vi "LED XControl Scroll.vi"(9 "Single pass?":bool, 10 "LEDDisplay":refnum<vi>, 11 "String":string="The Software is the Instrument     ") -> ()   [LabVIEW 2012, in "LED Display.xctl"]
doc: "This VI will control scrolling the XControl LED and displaying the string on LED Screen"
uses:
  LED Display.xctl
panel:
  # "This is the actual background task VI. It is reentrant and multiple clones of this VI may exist in memory, one for each of the LED XControls."
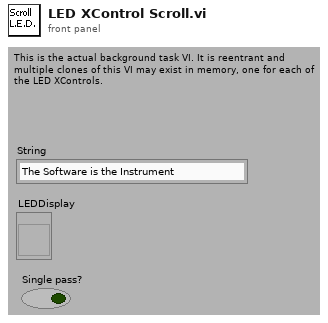
[diagram p1: front panel]
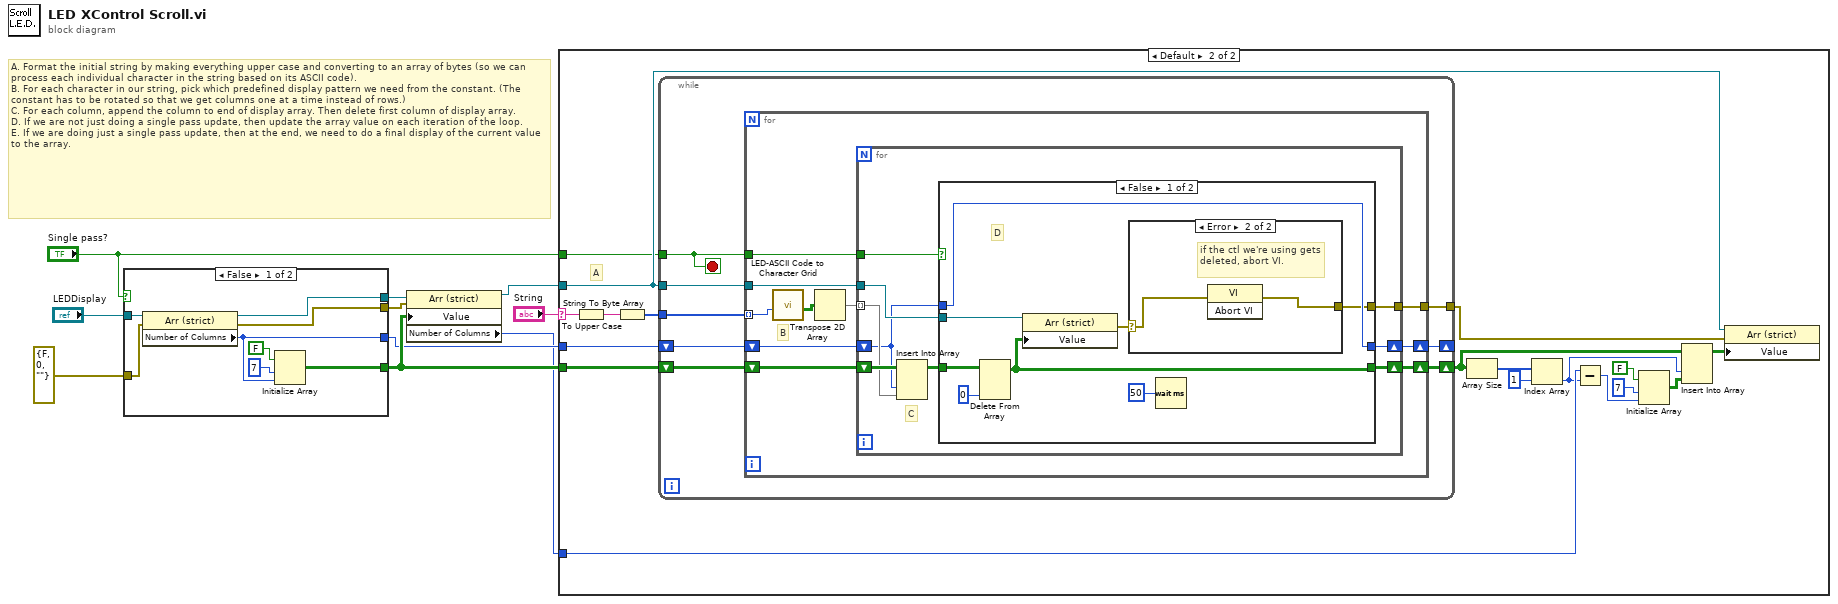
[diagram p0: block diagram]
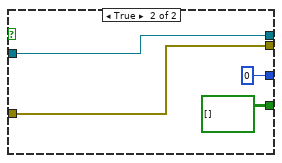
[diagram p2: hidden frame]
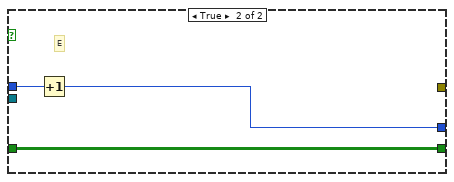
[diagram p5: hidden frame]
diagram:
  # "A. Format the initial string by making everything upper case and converting to an array of bytes (so we can process each individual character in the string based on its ASCII code).\nB. For each character in our string, pick which predefined display pattern we need from the constant. (The constant has to be rotated so that we get columns one at a time instead of rows.)\nC. For each column, append the column to end of display array. Then delete first column of display array.\nD. If we are not just doing a single pass update, then update the array value on each iteration of the loop.\nE. If we are doing just a single pass update, then at the end, we need to do a final display of the current value to the array."
  n1 = case shown="False" "Single pass?" {
    tunnel: "LEDDisplay" -> [w18 w22]
    tunnel: [w17 w22] -> w8
    tunnel: [w16 bool[][] []] -> w7
    tunnel: [w13 u32 0 ("Number of Columns")] -> w4
    tunnel: [w12 w19] -> w2
    tunnel: errorcluster {"status"=FALSE, "code"=0, "source"=""} ("error out") -> [w11 w19]
    frame False {
      n2 = property class="Arr (strict)"(reference=w18, error in=w11) -> (reference out=w17:refnum<vi>, error out=w12:errorcluster, "Number of Columns"=w13:u32)
      n3 = Initialize Array(FALSE ("Boolean"), 7 ("dimension size"), w13) -> (w16:bool[][])
    }
    frame True {
    }
  }
  n4 = property class="Arr (strict)"(reference=w8, error in=w2, "Value"=w7) -> (reference out=w6:refnum<vi>, "Number of Columns"=w3:u32)  [unwired: 1 out]
  n5 = case shown="Default" "String" {
    selector: "String" -> [_ w39]
    tunnel: w6 -> [_ w37]
    tunnel: w7 -> [_ w38]
    tunnel: "Single pass?" -> [_ w36]
    tunnel: w4 -> [_ w35]
    tunnel: w3 -> [_ w32]
    frame "" {
      # "do nothing for empty string."
    }
    frame Default {
      # "A"
      n6 = To Upper Case(1:w39) -> (0:w24:string)
      n7 = String To Byte Array(string=w24) -> (unsigned byte array=w40:u8[])
      n8 = while {
        tunnel: w40 -> [w48]
        shift-right: [w46] -> w26
        shift-left: w38 -> [w47]
        tunnel: w37 -> [w45]
        tunnel: w36 -> [w44]
        shift-right: [w42] -> _
        shift-left: w35 -> [w43]
        tunnel: [w41] -> w23
        stop <- w44 stop-if-true
        n9 = for {
          shift-right: [w58] -> w46
          shift-left: w47 -> [w57]
          tunnel: w48 -> [w50] mode=indexing
          tunnel: w45 -> [w54]
          tunnel: w44 -> [w53]
          shift-right: [w51] -> w42
          shift-left: w43 -> [w52]
          tunnel: [w49] -> w41
          # "B"
          n10 = call "LED-ASCII Code to Character Grid.vi"("ASCII Value"=w50) -> ("Character Grid"=w56:bool[][])  [unwired: 10 in]
          n11 = Transpose 2D Array(2D array=w56) -> (transposed array=w55:bool[][])
          n12 = for {
            shift-right: [w62] -> w58
            shift-left: w57 -> [w65]
            tunnel: w55 -> [w64] mode=indexing
            tunnel: w54 -> [w67]
            tunnel: w53 -> [w66]
            shift-right: [w60] -> w51
            shift-left: w52 -> [w61]
            tunnel: [w59] -> w49
            # "C"
            n13 = Insert Into Array(array=w65, index (col)=w61, new element=w64) -> (w63:bool[][])  [unwired: 1 in]
            n14 = case shown="False" w66 {
              tunnel: w67 -> [w74 _]
              tunnel: w63 -> [w71 w81]
              tunnel: [w70 w81] -> w62
              tunnel: w61 -> [w69 w80]
              tunnel: [w69 w79] -> w60
              tunnel: [w68 _] -> w59
              frame False {
                # "D"
                n15 = Delete From Array(array=w71, index (col)=0 ("Disabled Index (col)")) -> (array with subset deleted=w70:bool[][])  [unwired: 2 in, 1 out]
                n16 = property class="Arr (strict)"(reference=w74, "Value"=w70) -> (error out=w73:errorcluster)  [unwired: 1 in, 1 out]
                n17 = case shown="Error" w73 {
                  selector: w73 -> [w76 w78]
                  tunnel: [w76 w77] -> w68
                  frame No Error {
                  }
                  frame Error {
                    # "if the ctl we're using gets deleted, abort VI."
                    n18 = invoke class="VI" method="Abort VI"(error in=w78) -> (error out=w77:errorcluster)  [unwired: 2 in, 2 out]
                  }
                }
                n19 = Wait (ms)(milliseconds to wait=u32 50) -> ()  [unwired: 1 out]
              }
              frame True {
                # "E"
                n20 = Increment(x=w80) -> (x+1=w79:u32)
              }
            }
          }
        }
      }
      n21 = Array Size(array=w26) -> (size(s)=w34:i32[])
      n22 = Index Array(array=w34, index=1) -> (element=w28:i32)
      n23 = Subtract(x=w32, y=w28) -> (x-y=w31:u32)
      n24 = Initialize Array(FALSE ("replace all? (F)"), 7 ("dimension size"), w31) -> (w27:bool[][])
      n25 = Insert Into Array(array=w26, index (col)=w28, new element=w27) -> (w25:bool[][])  [unwired: 1 in]
      n26 = property class="Arr (strict)"(reference=w37, error in=w23, "Value"=w25) -> ()  [unwired: 2 out]
    }
  }
